vi "Unbenannt 3.vi"() -> ()   [LabVIEW 2013]
uses:
  classes/Datastructure/Report/Report.lvclass
  classes/Datastructure/Test/Test.lvclass
  classes/Datastructure/Segment/Segment.lvclass
  classes/Datastructure/Image/img.lvclass
  classes/Datastructure/Setup/Setup.lvclass
  classes/Datastructure/Device/Device.lvclass
  Main/controls/Data.ctl
  Main/controls/State.ctl
  classes/Devices/emTestCWS500N/EMTestCWS500N.lvclass
  classes/Devices/CEG4500/CEG4500.lvclass
  classes/Devices/Tektronix RSA5106A/Tektronix RSA5106A.lvclass
panel:
  in  "gelesen von XML":string(tree)
  in  "gelesen vom Baum":string(tree)
  out "Fehler (Ausgang)":errorcluster
  in  "gelesen von Datenstruktur":string(tree)
  out "Report (Ausgang)":refnum<class "Report.lvclass">
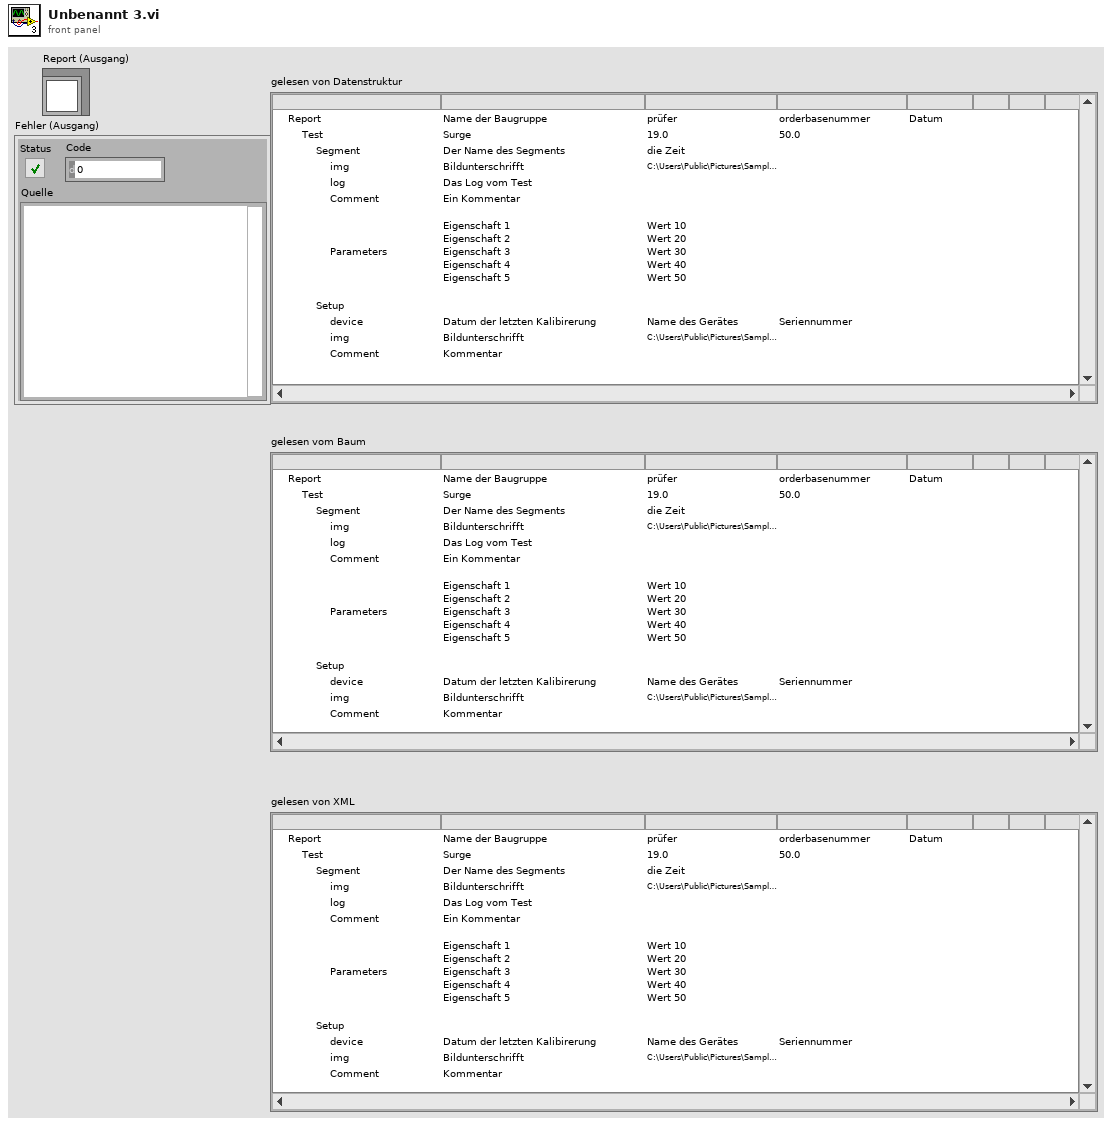
[diagram p1: front panel]
types:
  T1 = typedef "Data.ctl" = cluster{"Report.lvclass":refnum<class "Report.lvclass">, "test":string, "Initial State":T2, "test ID":i32, "parameter":string[][], "EMTestCWS500N.lvclass":refnum<class "EMTestCWS500N.lvclass">, "CEG4500.lvclass":refnum<class "CEG4500.lvclass">, "Tektronix RSA5106A.lvclass":refnum<class "Tektronix RSA5106A.lvclass">, "erfolgreich":bool, "log":string}
  T2 = typedef "State.ctl" = enum16{"CDN Kalibrierung", "enter Report Parameters", "new Test", "Protokoll", "read Tree", "update Tree", "Fehler", "Initialize", "Störaussendung", "Burst", "ESD", "Surge", "Spannungseinbruch", "HF-Felder", "Wait for Event", "Exit"}
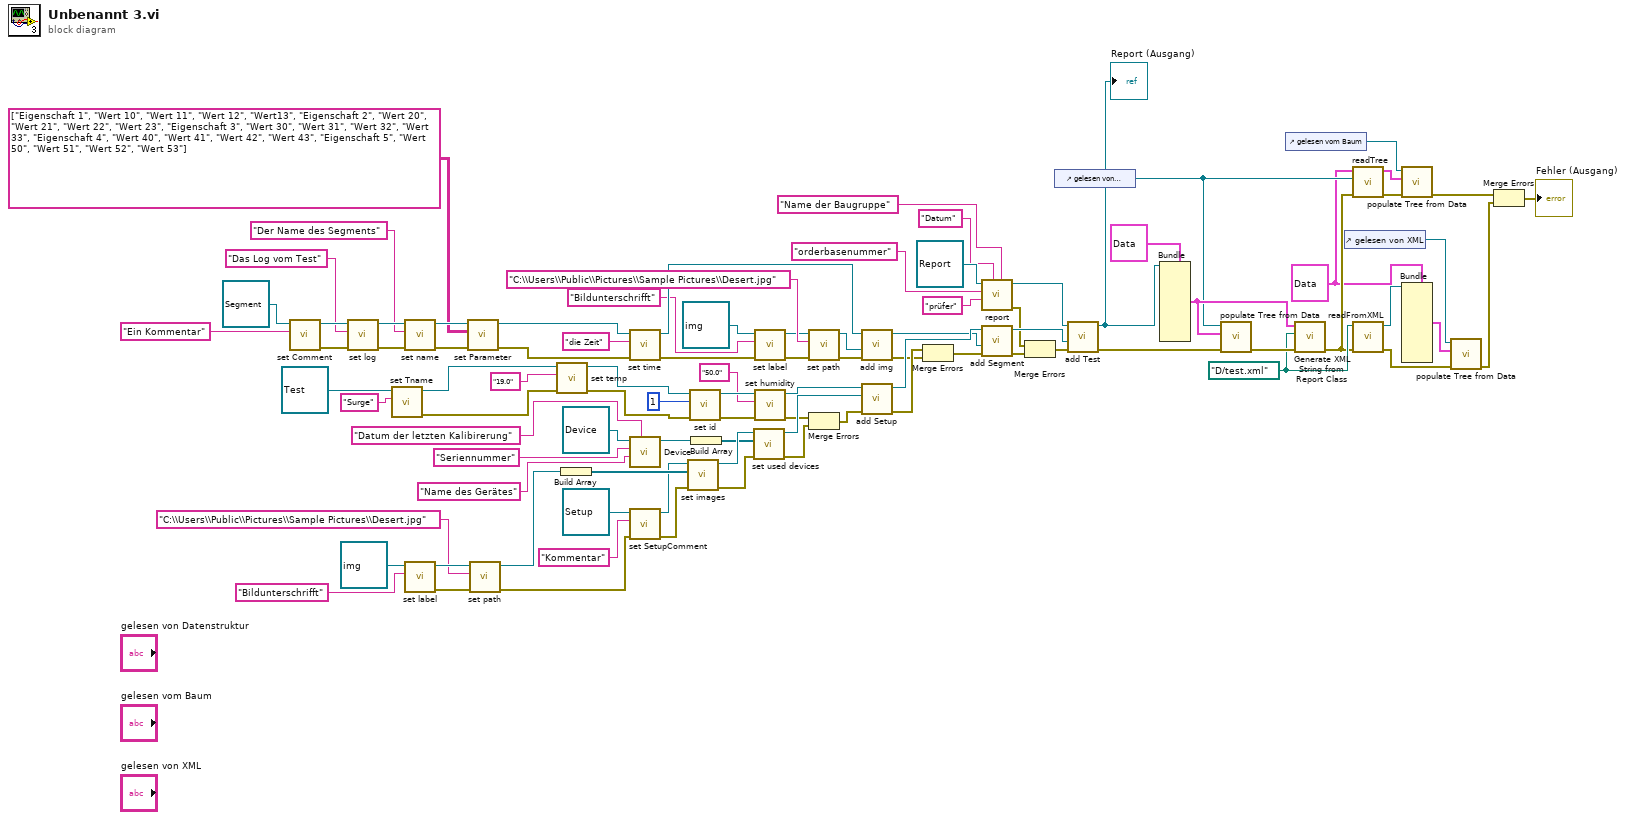
[diagram p0: block diagram]
diagram:
  w8 = T1 {"Report.lvclass"=refnum, "test"="", "Initial State"=enum."Initialize", "test ID"=0, "parameter"=[], "EMTestCWS500N.lvclass"=refnum, "CEG4500.lvclass"=refnum, "Tektronix RSA5106A.lvclass"=refnum, "erfolgreich"=FALSE, "log"=""} ("Data out (Eingang)")
  w10 = path "D:/test.xml" ("Dateipfad (Dialog verwenden)")
  n1 = call-dynamic "set Comment.vi"("Comment"="Ein Kommentar", "Segment (Eingang)"=refnum<class "Segment.lvclass"> refnum ("Segment.lvclass")) -> ("error out"=w65:errorcluster, "Segment (Ausgang)"=w72:refnum<class "Segment.lvclass">)  [unwired: 8 in]
  n2 = call-dynamic "set log.vi"("error in (no error)"=w65, "log"="Das Log vom Test", "Segment (Eingang)"=w72) -> ("error out"=w66:errorcluster, "Segment (Ausgang)"=w71:refnum<class "Segment.lvclass">)  [unwired: 7 in]
  n3 = call-dynamic "set Tname.vi"("name"="Surge", "Test (Eingang)"=refnum<class "Test.lvclass"> refnum ("Test.lvclass")) -> ("error out"=w82:errorcluster, "Test (Ausgang)"=w85:refnum<class "Test.lvclass">)  [unwired: 8 in]
  n4 = call-dynamic "set name.vi"("error in (no error)"=w66, "name"="Der Name des Segments", "Segment (Eingang)"=w71) -> ("error out"=w67:errorcluster, "Segment (Ausgang)"=w70:refnum<class "Segment.lvclass">)  [unwired: 7 in]
  n5 = call-dynamic "set label.vi"("label"="Bildunterschrifft", "img (Eingang)"=refnum<class "img.lvclass"> refnum ("img.lvclass")) -> ("error out"=w50:errorcluster, "img (Ausgang)"=w49:refnum<class "img.lvclass">)  [unwired: 8 in]
  n6 = call-dynamic "set Parameter.vi"("error in (no error)"=w67, "Parameter"=string[][] [["Eigenschaft 1", "Wert 10", "Wert 11", "Wert 12", "Wert13"], ["Eigenschaft 2", "Wert 20", "Wert 21", "Wert 22", "Wert 23"], ["Eigenschaft 3", "Wert 30", "Wert 31", "Wert 32", "Wert 33"], ["Eigenschaft 4", "Wert 40", "Wert 41", "Wert 42", "Wert 43"], ["Eigenschaft 5", "Wert 50", "Wert 51", "Wert 52", "Wert 53"]], "Segment (Eingang)"=w70) -> ("error out"=w68:errorcluster, "Segment (Ausgang)"=w69:refnum<class "Segment.lvclass">)  [unwired: 7 in]
  n7 = call-dynamic "set path.vi"("error in (no error)"=w50, "path"="C:\\Users\\Public\\Pictures\\Sample Pictures\\Desert.jpg", "img (Eingang)"=w49) -> ("error out"=w24:errorcluster, "img (Ausgang)"=w42:refnum<class "img.lvclass">)  [unwired: 7 in]
  n8 = call-dynamic "set temp.vi"("error in (no error)"=w82, "temp"="19.0", "Test (Eingang)"=w85) -> ("error out"=w81:errorcluster, "Test (Ausgang)"=w84:refnum<class "Test.lvclass">)  [unwired: 7 in]
  n9 = Build Array(w42) -> (w41:refnum<class "img.lvclass">[])
  n10 = call-dynamic "set time.vi"("error in (no error)"=w68, "time"="die Zeit", "Segment (Eingang)"=w69) -> ("error out"=w51:errorcluster, "Segment (Ausgang)"=w59:refnum<class "Segment.lvclass">)  [unwired: 7 in]
  n11 = call-dynamic "Device.vi"("last calibration"="Datum der letzten Kalibirerung", "Name"="Name des Gerätes", "serial"="Seriennummer", "Device Eingang"=refnum<class "Device.lvclass"> refnum ("Device.lvclass")) -> ("Device Ausgang"=w33:refnum<class "Device.lvclass">)  [unwired: 6 in, 1 out]
  n12 = call-dynamic "set SetupComment.vi"("error in (no error)"=w24, "Comment"="Kommentar", "Setup (Eingang)"=refnum<class "Setup.lvclass"> refnum ("Setup.lvclass")) -> ("error out"=w43:errorcluster, "Setup (Ausgang)"=w40:refnum<class "Setup.lvclass">)  [unwired: 7 in]
  n13 = call-dynamic "set images.vi"("error in (no error)"=w43, "images"=w41, "Setup (Eingang)"=w40) -> ("error out"=w39:errorcluster, "Setup (Ausgang)"=w38:refnum<class "Setup.lvclass">)  [unwired: 7 in]
  n14 = call-dynamic "set id.vi"("error in (no error)"=w81, "id"=1, "Test (Eingang)"=w84) -> ("error out"=w80:errorcluster, "Test (Ausgang)"=w83:refnum<class "Test.lvclass">)  [unwired: 7 in]
  n15 = Build Array(w33) -> (w32:refnum<class "Device.lvclass">[])
  n16 = call-dynamic "set used devices.vi"("error in (no error)"=w39, "used devices"=w32, "Setup (Eingang)"=w38) -> ("error out"=w28:errorcluster, "Setup (Ausgang)"=w31:refnum<class "Setup.lvclass">)  [unwired: 7 in]
  n17 = call-dynamic "set label.vi"("error in (no error)"=w51, "label"="Bildunterschrifft", "img (Eingang)"=refnum<class "img.lvclass"> refnum ("img.lvclass")) -> ("error out"=w52:errorcluster, "img (Ausgang)"=w55:refnum<class "img.lvclass">)  [unwired: 7 in]
  n18 = call-dynamic "set humidity.vi"("error in (no error)"=w80, "humidity"="50.0", "Test (Eingang)"=w83) -> ("error out"=w29:errorcluster, "Test (Ausgang)"=w74:refnum<class "Test.lvclass">)  [unwired: 7 in]
  n19 = call-dynamic "set path.vi"("error in (no error)"=w52, "path"="C:\\Users\\Public\\Pictures\\Sample Pictures\\Desert.jpg", "img (Eingang)"=w55) -> ("error out"=w53:errorcluster, "img (Ausgang)"=w54:refnum<class "img.lvclass">)  [unwired: 7 in]
  n20 = Merge Errors(w29, w28) -> (w27:errorcluster)
  n21 = call-dynamic "add img.vi"("error in (no error)"=w53, "img.lvclass"=w54, "Segment (Eingang)"=w59) -> ("error out"=w25:errorcluster, "Segment (Ausgang)"=w30:refnum<class "Segment.lvclass">)  [unwired: 6 in]
  n22 = call-dynamic "add Setup.vi"("error in (no error)"=w27, "Setup"=w31, "Test Eingang"=w74) -> ("error out"=w26:errorcluster, "Test Ausgang"=w87:refnum<class "Test.lvclass">)  [unwired: 7 in]
  n23 = Merge Errors(w26, w25) -> (w23:errorcluster)
  n24 = call-dynamic "report.vi"("Rname"="Name der Baugruppe", "date"="Datum", "pruefer"="prüfer", "obnr"="orderbasenummer", "Report in"=refnum<class "Report.lvclass"> refnum ("Report.lvclass")) -> ("error out"=w22:errorcluster, "Report out"=w92:refnum<class "Report.lvclass">)  [unwired: 5 in]
  n25 = call-dynamic "add Segment.vi"("error in (no error)"=w23, "Segment.lvclass"=w30, "Test Eingang"=w87) -> ("error out"=w21:errorcluster, "Test Ausgang"=w86:refnum<class "Test.lvclass">)  [unwired: 7 in]
  n26 = Merge Errors(w22, w21) -> (w20:errorcluster)
  n27 = control-ref of="gelesen von Datenstruktur"() -> (w14:refnum<vi>)
  n28 = call-dynamic "add Test.vi"("error in (no error)"=w20, "Test.lvclass"=w86, "Report (Eingang)"=w92) -> ("error out"=w16:errorcluster, "Report (Ausgang)"=w18:refnum<class "Report.lvclass">)  [unwired: 7 in]
  "Report (Ausgang)" <- w18
  n29 = Bundle(cluster=T1 {"Report.lvclass"=refnum, "test"="", "Initial State"=enum."Protokoll", "test ID"=0, "parameter"=[], "EMTestCWS500N.lvclass"=refnum, "CEG4500.lvclass"=refnum, "Tektronix RSA5106A.lvclass"=refnum, "erfolgreich"=FALSE, "log"=""} ("Data"), "Report.lvclass"=w18) -> (w17:T1)  [unwired: 9 in]
  n30 = call "populate Tree from Data.vi"("error in (no error)"=w16, "Data"=w17, "reference"=w14) -> ("error out"=w15:errorcluster)  [unwired: 6 in]
  n31 = control-ref of="gelesen vom Baum"() -> (w12:refnum<vi>)
  n32 = call "Generate XML String from Report Class.vi"("error in (no error)"=w15, "Dateipfad (Dialog verwenden)"=w10, "Data"=w17) -> ("Fehler (Ausgang)"=w9:errorcluster)  [unwired: 8 in]
  n33 = control-ref of="gelesen von XML"() -> (w5:refnum<vi>)
  n34 = call "readTree.vi"("Fehler (Eingang, kein Fehler)"=w9, "Tree ref"=w14, "Data out (Eingang)"=w8) -> ("error out"=w11:errorcluster, "Data out (Ausgang)"=w13:T1)  [unwired: 7 in]
  n35 = call "readFromXML.vi"("error in (no error)"=w9, "file path (use dialog)"=w10) -> ("error out"=w4:errorcluster, "Report (Ausgang)"=w7:refnum<class "Report.lvclass">)  [unwired: 8 in]
  n36 = call "populate Tree from Data.vi"("error in (no error)"=w11, "Data"=w13, "reference"=w12) -> ("error out"=w2:errorcluster)  [unwired: 6 in]
  n37 = Bundle(cluster=w8, "Report.lvclass"=w7) -> (w6:T1)  [unwired: 9 in]
  n38 = call "populate Tree from Data.vi"("error in (no error)"=w4, "Data"=w6, "reference"=w5) -> ("error out"=w3:errorcluster)  [unwired: 6 in]
  n39 = Merge Errors(w2, w3) -> (→"Fehler (Ausgang)":errorcluster)
